vi "Time stamp to time string.vi"(8 "error in (no error)":errorcluster, 10 "Time Stamp":timestamp, 11 "OLE DB Timestamp in":refnum<class "OLE DB Timestamp.lvclass">) -> (0 "error out":errorcluster, 2 "String":string, 3 "OLE DB Timestamp out":refnum<class "OLE DB Timestamp.lvclass">)   [LabVIEW 2020, in "Basic Columns.lvlib" / "OLE DB Timestamp.lvclass"]
uses:
  OLE DB Timestamp.lvclass
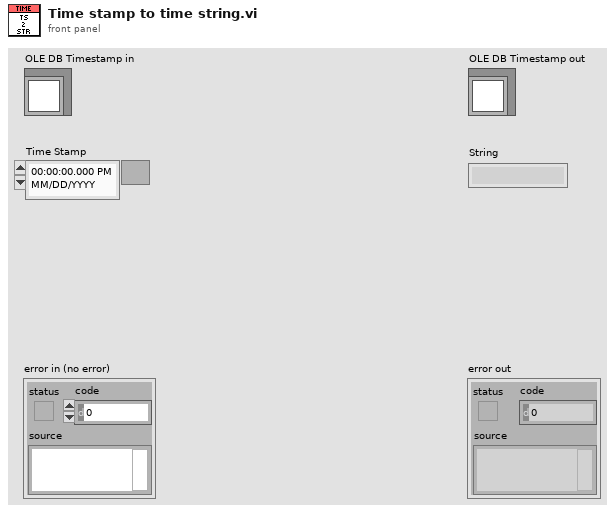
[diagram p1: front panel]
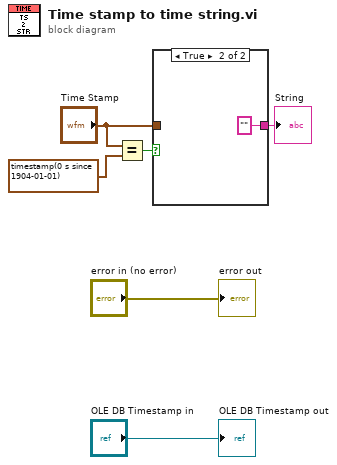
[diagram p0: block diagram]
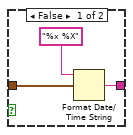
[diagram p2: hidden frame]
diagram:
  n1 = Equal?(x="Time Stamp", y=timestamp(0 s since 1904-01-01) ("Time Stamp")) -> (x = y?=w1:bool)
  n2 = case shown="True" w1 {
    tunnel: [w9 "" ("date/time string")] -> w5
    tunnel: "Time Stamp" -> [w7 _]
    frame False {
      n3 = Format Date/Time String(time format string (%c)="%x %X" ("format string"), seconds (now)=w7) -> (date/time string=w9:string)  [unwired: 1 in]
    }
    frame True {
    }
  }
  "String" <- w5
  "error out" <- "error in (no error)"
  "OLE DB Timestamp out" <- "OLE DB Timestamp in"
